vi "Configure Digital Pin Direction.vi"(8 "error in (no error)":errorcluster, 10 "Pin Direction":T1(array[cluster]), 11 "VISA resource name":refnum<visa-resource-name>) -> (0 "error in (no error) 2":errorcluster, 3 "VISA resource name 2":refnum<visa-resource-name>)   [LabVIEW 2020, in "BDAQ-6104.lvlib"]
uses:
  <instrlib>/BDAQ-6104/BDAQ-6104.lvlib
panel:
  # "Input"
  # "Output"
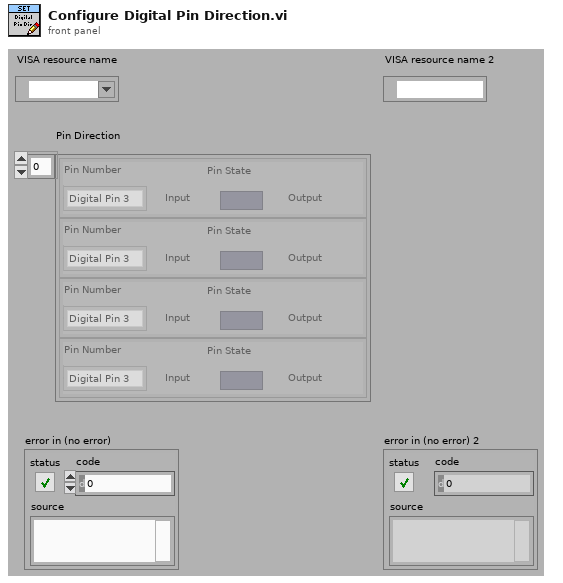
[diagram p1: front panel]
types:
  T1 = cluster{"Pin Number":enum16{"Digital Pin 0", "Digital Pin 1", "Digital Pin 2", "Digital Pin 3"}, "Pin State":bool}[]
  T2 = enum16{"Digital Pin 0", "Digital Pin 1", "Digital Pin 2", "Digital Pin 3"}
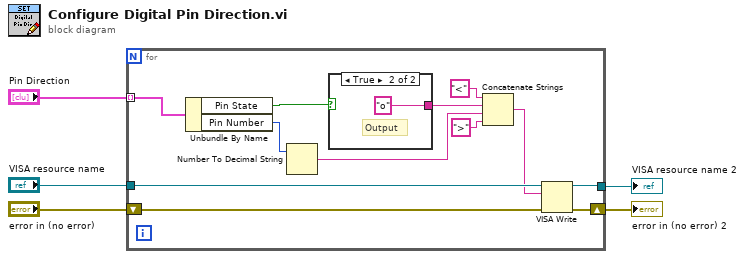
[diagram p0: block diagram]
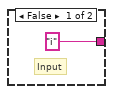
[diagram p2: hidden frame]
diagram:
  n1 = for {
    tunnel: "VISA resource name" -> [w17]
    tunnel: "Pin Direction" -> [w15] mode=indexing
    tunnel: [w7] -> w2
    shift-right: [w6] -> w1
    shift-left: "error in (no error)" -> [w16]
    n2 = Unbundle By Name(w15) -> ("Pin State"=w13:bool, "Pin Number"=w11:T2)
    n3 = Number To Decimal String(number=w11) -> (decimal integer string=w10:string)  [unwired: 1 in]
    n4 = case shown="True" w13 {
      tunnel: ["i" "o"] -> w12
      frame False {
        # "Input"
      }
      frame True {
        # "Output"
      }
    }
    n5 = Concatenate Strings("<", w12, w10, ">" ("string")) -> (w8:string)
    n6 = VISA Write(VISA resource name=w17, write buffer=w8, error in (no error)=w16) -> (VISA resource name out=w7:refnum<visa-resource-name>, error out=w6:errorcluster)  [unwired: 1 out]
  }
  "VISA resource name 2" <- w2
  "error in (no error) 2" <- w1
